vi "Get Clone Number.vi"() -> (0 "caller clone#":i32)   [LabVIEW 2020, in "NI_TargetHelper.lvlib"]
uses:
  <vilib>/TargetSupport/NI_TargetHelper/NI_TargetHelper.lvlib
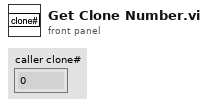
[diagram p1: front panel]
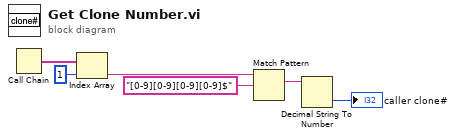
[diagram p0: block diagram]
diagram:
  n1 = Call Chain() -> (call chain=w6:string[])
  n2 = Index Array(array=w6, index=1) -> (element=w4:string)
  n3 = Match Pattern(string=w4, regular expression="[0-9][0-9][0-9][0-9]$") -> (match substring=w2:string)  [unwired: 1 in, 3 out]
  n4 = Decimal String To Number(string=w2) -> (number=→"caller clone#":i32)  [unwired: 2 in, 1 out]
